vi "FG - FilePathnames.vi"(4 "action (Get)":T2=enum."Get", 5 "FilePaths in":T1) -> (1 "RunTimeSys?":bool, 2 "FilePaths out":T1={"RunTimeSys?"=FALSE, "AppFolder"=path "C:/Projects/InfiniRel/IHS", "ExecutablePath"=path "<NONE>", "ConfigFolder"=path "C:/IHS/Config", "DataLogFolder"=path "C:/IHS/DataLog", "SystemLogFolder"=path "C:/IHS/SystemLog", "SeqFolder"=path "C:/IHS/SeqFolder", "MainStartupPathname"=path "C:/Projects/InfiniRel/IHS/Source/Application/Process_Application.vi", "MainUIPathname"=path "C:/Projects/InfiniRel/IHS/Source/Main/IHS_MainUI.vi", "SystemEventsFile"=path "C:/IHS/SystemLog/SystemEvents.txt", "SeqEventsFile"=path "C:/IHS/SeqFolder/SeqEvents.txt", "Config SettingsFile"=path "C:/IHS/Config/IHS_Config.xml", "DAQ IOConfigFile"=path "C:/IHS/Config/IOConfig.xml", "SystemSimulation"=FALSE})   [LabVIEW 2019]
doc: "Developed by Kevin Thompson\nkevin@thompsonengineering.net\n\nCopyright 2018-2020\nThompson Engineering, LLC"
uses:
  Source/Common/Startup/GBL System.vi
  <userlib>/_OpenG.lib/file/file.llb/Build Path - Traditional__ogtk.vi
  Source/Common/DataTypes/TD GetSet ActionSelect--enum.ctl
  Source/Common/Startup/TD Pathnames--cluster.ctl
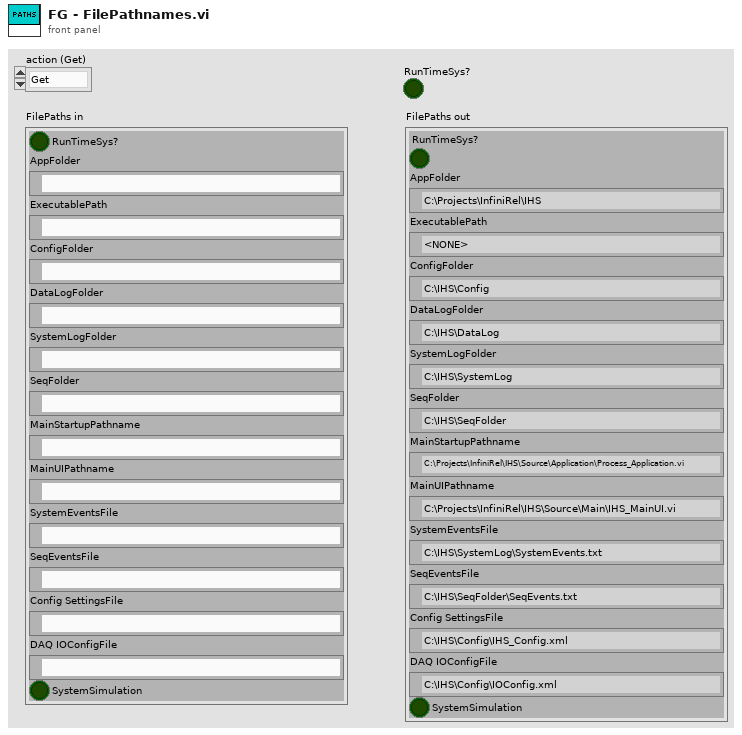
[diagram p1: front panel]
types:
  T1 = typedef "TD Pathnames--cluster.ctl" = cluster{"RunTimeSys?":bool, "AppFolder":path, "ExecutablePath":path, "ConfigFolder":path, "DataLogFolder":path, "SystemLogFolder":path, "SeqFolder":path, "MainStartupPathname":path, "MainUIPathname":path, "SystemEventsFile":path, "SeqEventsFile":path, "Config SettingsFile":path, "DAQ IOConfigFile":path, "SystemSimulation":bool}
  T2 = typedef "TD GetSet ActionSelect--enum.ctl" = enum16{"Init", "Get", "Set"}
  T3 = typedef "Startup INI Data--cluster.ctl" = cluster{"ConfigFolder":path, "DataLogFolder":path, "SystemLogFolder":path, "SequenceFolder":path, "ApplicationStartup":string, "MainUI":string, "AppConfigFilename":string, "IOConfigFilename":string, "SystemSimulation":bool}
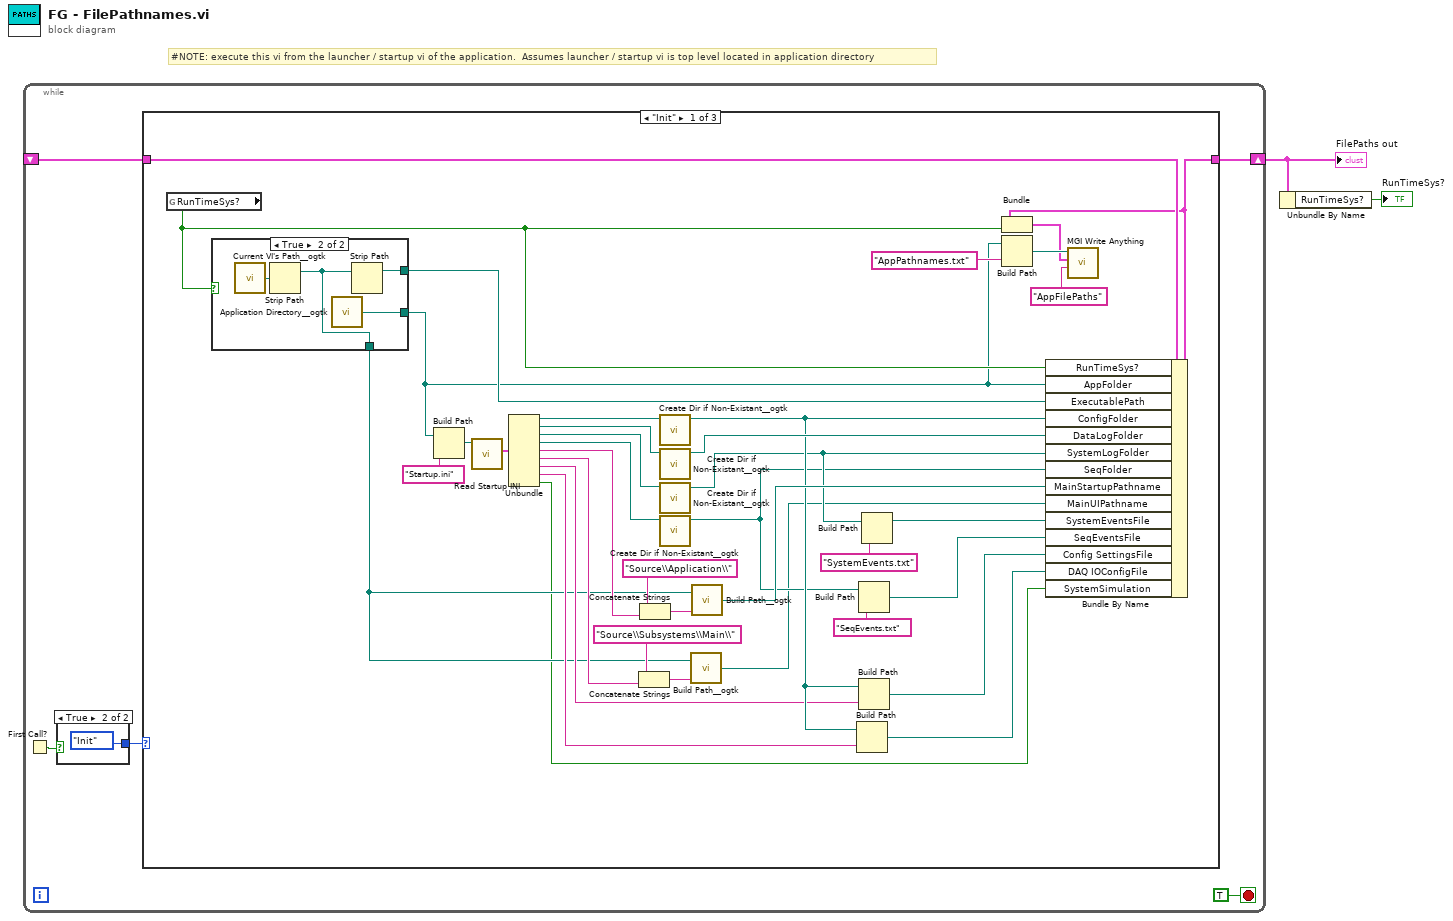
[diagram p0: block diagram]
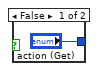
[diagram p2: hidden frame]
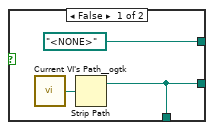
[diagram p3: hidden frame]
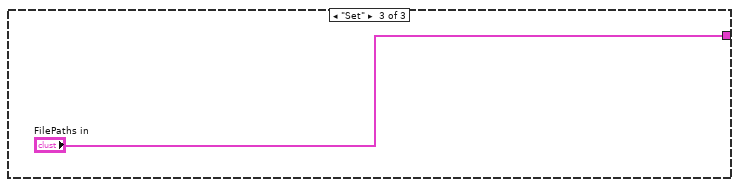
[diagram p5: hidden frame]
diagram:
  # "#NOTE: execute this vi from the launcher / startup vi of the application.  Assumes launcher / startup vi is top level located in application directory"
  n1 = while {
    shift-right: [w6] -> w2
    shift-left: _ -> [w5]
    stop <- TRUE stop-if-true
    n2 = First Call?() -> (First Call?: T/F=w3:bool)
    n3 = case shown="True" w3 {
      tunnel: ["action (Get)" TD_GetSet_ActionSelect--enum."Init" ("action (Get)")] -> w7
      frame False {
      }
      frame True {
      }
    }
    n4 = case shown="\"Init\"" w7 {
      tunnel: [w43 w55 "FilePaths in"] -> w6
      tunnel: w5 -> [w47 w55 _]
      frame "Init" {
        n5 = global read "GBL System.vi" "RunTimeSys?"() -> (w40:bool)
        n6 = case shown="True" w40 {
          tunnel: [w48 w54] -> w36
          tunnel: [path "<NONE>" ("Parent Directory (+ Relative)") w52] -> w41
          tunnel: [w48 w51] -> w12
          frame False {
            n7 = call <userlib>:"Current VI's Path__ogtk.vi"() -> ("Current VI's Path (+ Relative)"=w49:path)  [unwired: 1 in]
            n8 = Strip Path(path=w49) -> (stripped path=w48:path)  [unwired: 1 out]
          }
          frame True {
            n9 = call <userlib>:"Current VI's Path__ogtk.vi"() -> ("Current VI's Path (+ Relative)"=w53:path)  [unwired: 1 in]
            n10 = Strip Path(path=w53) -> (stripped path=w51:path)  [unwired: 1 out]
            n11 = call <userlib>:"Application Directory__ogtk.vi"() -> ("Application Directory (+ Relative)"=w54:path)  [unwired: 1 in]
            n12 = Strip Path(path=w51) -> (stripped path=w52:path)  [unwired: 1 out]
          }
        }
        n13 = Build Path(base path=w36, name or relative path="Startup.ini") -> (appended path=w37:path)
        n14 = call "Read Startup INI.vi"("Startup INI file"=w37) -> ("Startup INI"=w34:T3)  [unwired: 8 in, 2 out]
        n15 = Unbundle(w34) -> ("ConfigFolder"=w33:path, "DataLogFolder"=w32:path, "SystemLogFolder"=w31:path, "SequenceFolder"=w20:path, "ApplicationStartup"=w18:string, "MainUI"=w14:string, "AppConfigFilename"=w16:string, "IOConfigFilename"=w17:string, "SystemSimulation"=w10:bool)
        n16 = Concatenate Strings("Source\\Subsystems\\Main\\" ("string"), w14) -> (w15:string)
        n17 = Concatenate Strings("Source\\Application\\" ("string"), w18) -> (w25:string)
        n18 = call <userlib>:"Create Dir if Non-Existant__ogtk.vi"("Directory Path"=w33) -> ("dup Directory Path"=w24:path)  [unwired: 8 in, 2 out]
        n19 = call <userlib>:"Create Dir if Non-Existant__ogtk.vi"("Directory Path"=w32) -> ("dup Directory Path"=w30:path)  [unwired: 8 in, 2 out]
        n20 = call <userlib>:"Create Dir if Non-Existant__ogtk.vi"("Directory Path"=w31) -> ("dup Directory Path"=w21:path)  [unwired: 8 in, 2 out]
        n21 = call <userlib>:"Create Dir if Non-Existant__ogtk.vi"("Directory Path"=w20) -> ("dup Directory Path"=w19:path)  [unwired: 8 in, 2 out]
        n22 = call-poly <userlib>:"Build Path__ogtk.vi"("name or relative path"=w15, "base path"=w12) -> ("appended path"=w11:path)
        n23 = call-poly <userlib>:"Build Path__ogtk.vi"("name or relative path"=w25, "base path"=w12) -> ("appended path"=w27:path)
        n24 = Build Path(base path=w24, name or relative path=w17) -> (appended path=w28:path)
        n25 = Build Path(base path=w19, name or relative path="SeqEvents.txt") -> (appended path=w22:path)
        n26 = Build Path(base path=w24, name or relative path=w16) -> (appended path=w29:path)
        n27 = Build Path(base path=w21, name or relative path="SystemEvents.txt") -> (appended path=w38:path)
        n28 = Build Path(base path=w36, name or relative path="AppPathnames.txt") -> (appended path=w46:path)
        n29 = Bundle By Name(cluster=w47, "RunTimeSys?"=w40, "AppFolder"=w36, "ExecutablePath"=w41, "ConfigFolder"=w24, "DataLogFolder"=w30, "SystemLogFolder"=w21, "SeqFolder"=w19, "MainStartupPathname"=w27, "MainUIPathname"=w11, "SystemEventsFile"=w38, "SeqEventsFile"=w22, "Config SettingsFile"=w29, "DAQ IOConfigFile"=w28, "SystemSimulation"=w10) -> (w43:T1)
        n30 = Bundle("FilePaths in"=w43, "RunTimeSys?"=w40) -> (w42:cluster{"FilePaths in":T1, "RunTimeSys?":bool})  [unwired: 1 in]
        n31 = call <userlib>:"MGI Write Anything.vi"("Section Name (Name of \"Anything\")"="AppFilePaths" ("Section Name (Name of \"Anything\")"), "Anything"=w42, "Path (dialog)"=w46) -> ()  [unwired: 6 in, 3 out]
      }
      frame "Get", Default {
      }
      frame "Set" {
      }
    }
  }
  "FilePaths out" <- w2
  n32 = Unbundle By Name(w2) -> ("RunTimeSys?"=→"RunTimeSys?":bool)
